vi "ex4-2.vi"() -> ()   [LabVIEW 2019]
panel:
  out "LED 3":bool
  out "LED 2":bool
  out "LED1":bool
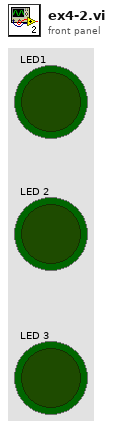
[diagram p1: front panel]
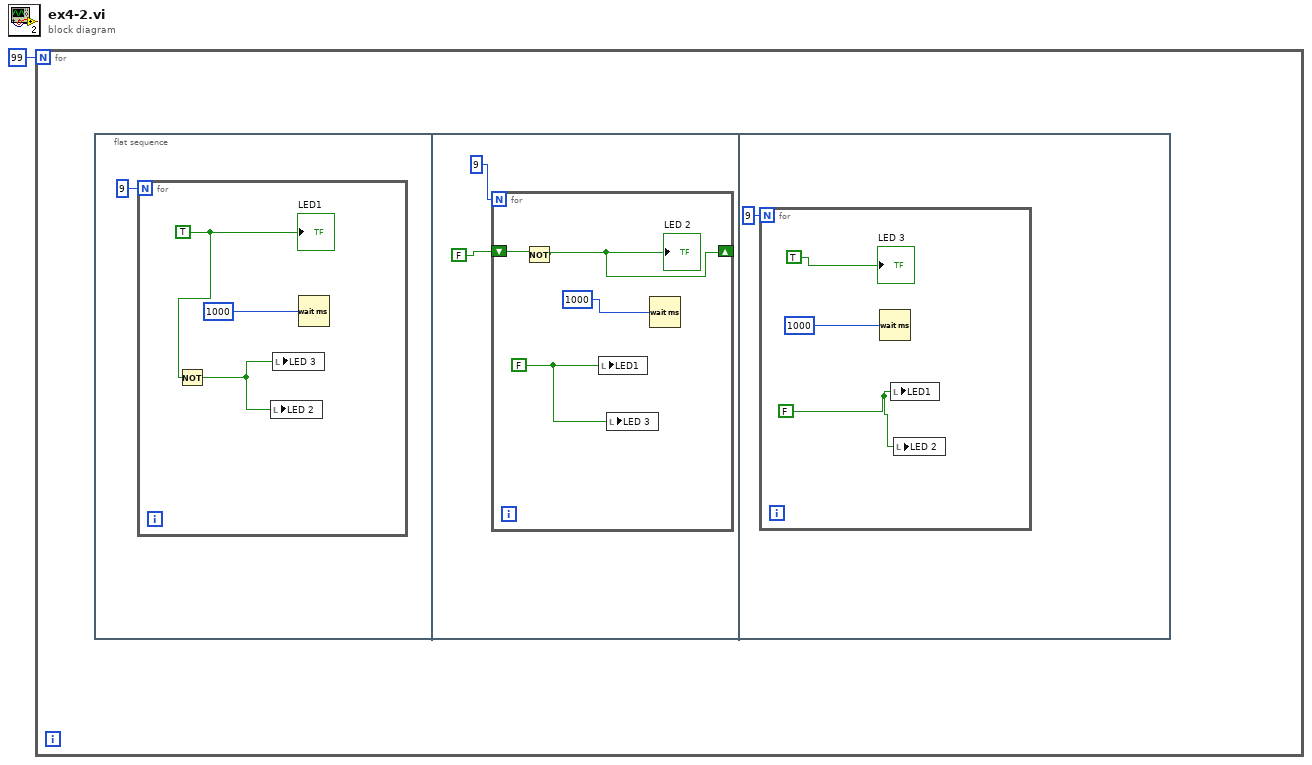
[diagram p0: block diagram]
diagram:
  n1 = for {
    N: 99 -> [_]
    n2 = flat-sequence {
      frame #0 {
        n3 = for {
          N: 9 -> [_]
          w3 = TRUE
          n4 = Not(x=w3) -> (.not. x?=w4:bool)
          n5 = local write "LED 2"(w4) -> ()
          n6 = local write "LED 3"(w4) -> ()
          n7 = Wait (ms)(milliseconds to wait=1000) -> ()  [unwired: 1 out]
          "LED1" <- w3
        }
      }
      frame #1 {
        n8 = for {
          N: 9 -> [_]
          shift-right: [w10] -> _
          shift-left: FALSE -> [w11]
          w8 = FALSE ("Boolean")
          n9 = Not(x=w11) -> (.not. x?=w10:bool)
          "LED 2" <- w10
          n10 = local write "LED1"(w8) -> ()
          n11 = local write "LED 3"(w8) -> ()
          n12 = Wait (ms)(milliseconds to wait=1000) -> ()  [unwired: 1 out]
        }
      }
      frame #2 {
        n13 = for {
          N: 9 -> [_]
          w13 = FALSE ("Boolean")
          n14 = Wait (ms)(milliseconds to wait=1000) -> ()  [unwired: 1 out]
          n15 = local write "LED1"(w13) -> ()
          n16 = local write "LED 2"(w13) -> ()
          "LED 3" <- TRUE
        }
      }
    }
  }
